vi "[Property] Fahrenheit Mode Read.vi"(4 "error in (no error)":errorcluster, 6 "Container State":T2, 7 "Display State In":T1) -> (0 "error out":errorcluster, 2 "Value":bool, 3 "Display State Out":T1)   [LabVIEW 2012, in "Simple Dual Mode Thermometer XControl.xctl"]
doc: "This VI handles the Fahrenheit? Read property as part of the Simple Dual Mode Thermometer XControl."
uses:
  Simple Dual Mode Thermometer XControl.xctl
  <vilib>/_xctls/Container State.ctl
  Simple Dual Mode Thermometer State.ctl
  <vilib>/_xctls/XControlSupport.lvlib
panel:
  # "See block diagram"
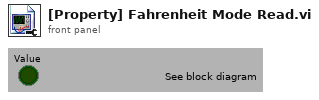
[diagram p1: front panel]
types:
  T1 = typedef "Simple Dual Mode Thermometer XControl.xctl/Simple Dual Mode Thermometer State.ctl" = cluster{"Fahrenheit":bool}
  T2 = typedef "XControlSupport.lvlib/Container State.ctl" = cluster{"Indicator?":bool, "Run Mode?":bool, " Refnum":refnum<vi>}
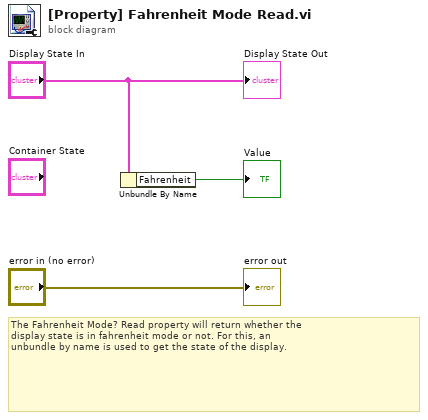
[diagram p0: block diagram]
diagram:
  # "The Fahrenheit Mode? Read property will return whether the \ndisplay state is in fahrenheit mode or not. For this, an\nunbundle by name is used to get the state of the display."
  n1 = Unbundle By Name("Display State In") -> ("Fahrenheit"=→"Value":bool)
  "error out" <- "error in (no error)"
  "Display State Out" <- "Display State In"
